vi "Value_JSON.vi"(0 "Data JSON":string, 5 "Type":string, 7 "Size data":string, 9 "Hexa":string, 11 "error in":errorcluster) -> (4 "Value_string":string, 8 "Hexa value":string, 15 "error IO":errorcluster)   [LabVIEW 2021]
uses:
  <vilib>/JDP Science/JSONtext/String Subset.vi
  <vilib>/JDP Science/JSONtext/support/Strip Quotes and Unescape.vi
  <vilib>/JDP Science/JSONtext/support/Unescape JSON string.vi
  <vilib>/JDP Science/JSONtext/Parsing/Parse Full Path or Item Name.vi
  <vilib>/JDP Science/JSONtext/Offset/Find Item Locations by Path.vi
  <vilib>/JDP Science/JSONtext/JSONtext.lvlib
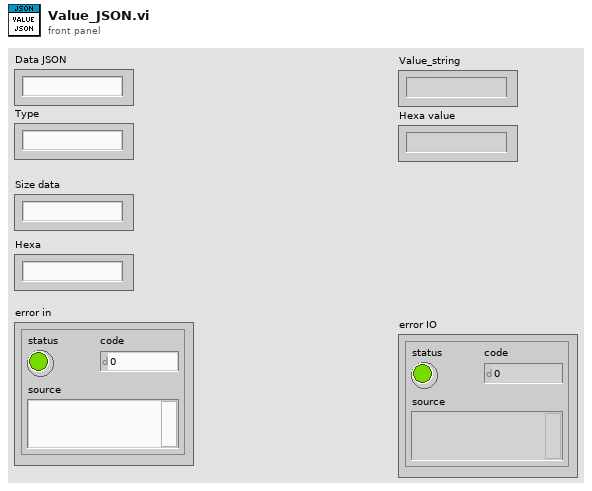
[diagram p1: front panel]
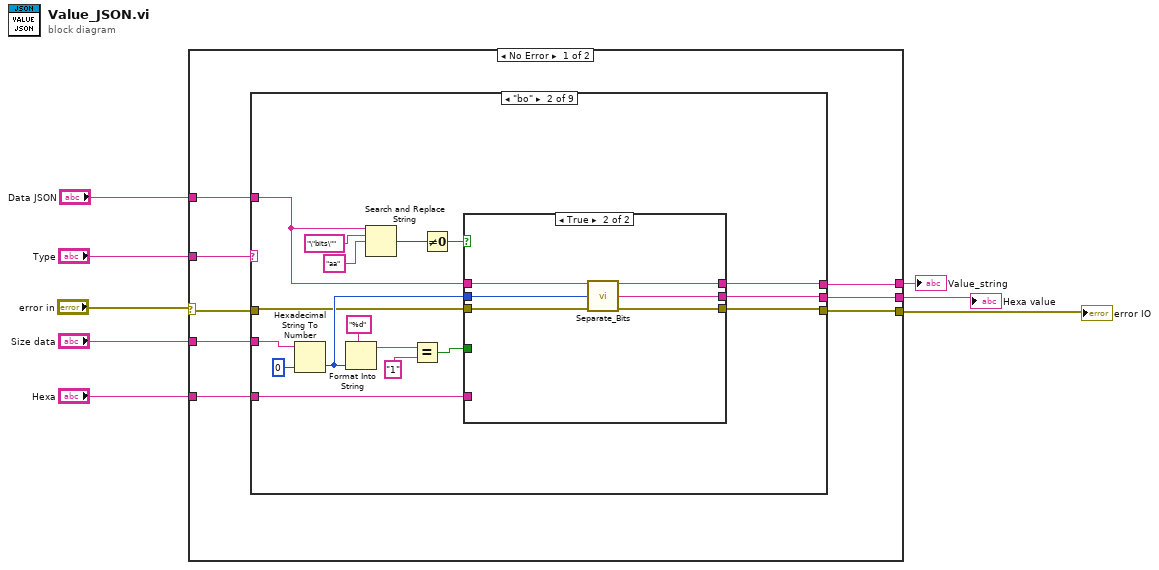
[diagram p0: block diagram]
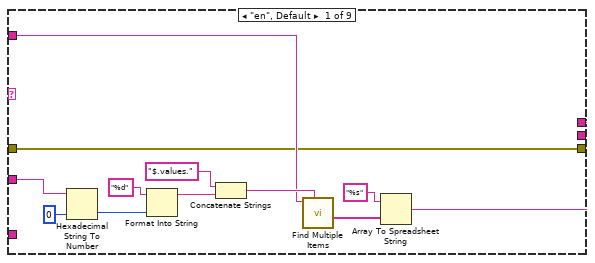
[diagram p2: hidden frame]
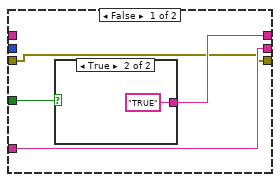
[diagram p3: hidden frame]
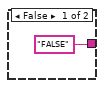
[diagram p4: hidden frame]
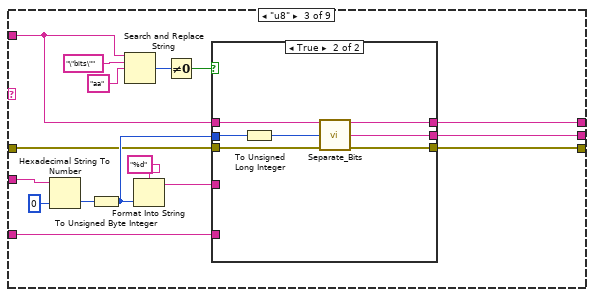
[diagram p5: hidden frame]
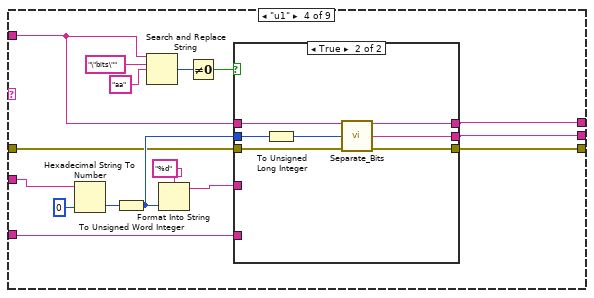
[diagram p7: hidden frame]
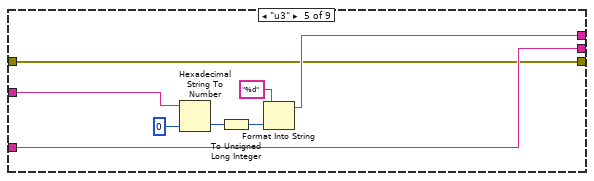
[diagram p9: hidden frame]
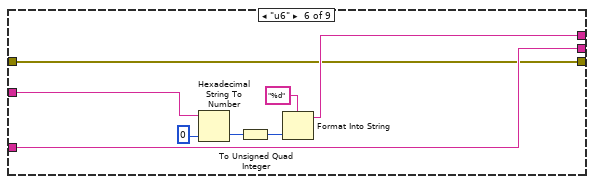
[diagram p10: hidden frame]
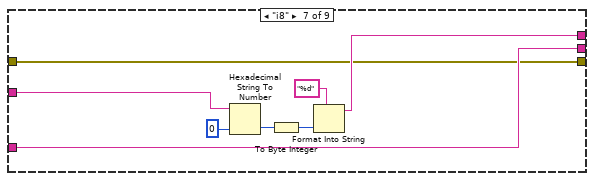
[diagram p11: hidden frame]
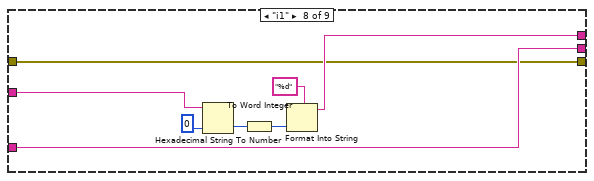
[diagram p12: hidden frame]
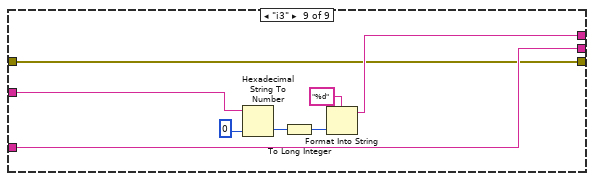
[diagram p13: hidden frame]
diagram:
  n1 = case shown="No Error" "error in" {
    selector: "error in" -> [w12 w150]
    tunnel: "Data JSON" -> [w16 _]
    tunnel: "Size data" -> [w15 _]
    tunnel: "Type" -> [w14 _]
    tunnel: "Hexa" -> [w13 _]
    tunnel: [w11 w150] -> w1
    tunnel: [w10 _] -> w2
    tunnel: [w9 _] -> w3
    frame No Error {
      n2 = case shown="\"bo\"" w14 {
        tunnel: w15 -> [w22 w44 w66 w89 w113 w121 w129 w137 w145]
        tunnel: [w19 w34 w64 w87 w112 w120 w128 w136 w144] -> w9
        tunnel: [_ w33 w61 w86 w111 w119 w127 w135 w143] -> w10
        tunnel: w13 -> [_ w32 w62 w90 w111 w119 w127 w135 w143]
        tunnel: w16 -> [w18 w36 w63 w88 _ _ _ _ _]
        tunnel: w12 -> [w17 w30 w59 w85 w110 w118 w126 w134 w142]
        tunnel: [w17 w29 w58 w84 w110 w118 w126 w134 w142] -> w11
        frame "en", Default {
          n3 = Hexadecimal String To Number(string=w22, default (0uL)=u32 0 ("default (0 U32)")) -> (number=w28:u32)  [unwired: 1 in, 1 out]
          n4 = Format Into String(format string="%d", w28) -> (resulting string=w25:string)  [unwired: 2 in, 1 out]
          n5 = Concatenate Strings("$.values." ("string"), w25) -> (w24:string)
          n6 = call <vilib>:"Find Multiple Items.vi"("$Path or Item Name"=w24, "JSON"=w18) -> ("<JSON>"=w20:string[])  [unwired: 6 in, 3 out]
          n7 = Array To Spreadsheet String(array=w20, 3:"%s" ("format string")) -> (spreadsheet string=w19:string)  [unwired: 1 in]
        }
        frame "bo" {
          n8 = Hexadecimal String To Number(string=w44, default (0uL)=u32 0 ("default (0 U32)")) -> (number=w31:u32)  [unwired: 1 in, 1 out]
          n9 = Format Into String(format string="%d", w31) -> (resulting string=w43:string)  [unwired: 2 in, 1 out]
          n10 = Search and Replace String(input string=w36, search string="\"bits\"", replace string="aa" ("replace string (\"\")")) -> (number of replacements=w38:i32)  [unwired: 5 in, 3 out]
          n11 = Equal?(x=w43, y="1") -> (x = y?=w35:bool)
          n12 = Not Equal To 0?(x=w38) -> (x != 0?=w37:bool)
          n13 = case shown="True" w37 {
            tunnel: [w48 w55] -> w34
            tunnel: w36 -> [_ w57]
            tunnel: [w47 w54] -> w33
            tunnel: w35 -> [w49 _]
            tunnel: w32 -> [w47 _]
            tunnel: w31 -> [_ w56]
            tunnel: w30 -> [w46 w53]
            tunnel: [w46 w52] -> w29
            frame False {
              n14 = case shown="True" w49 {
                tunnel: ["FALSE" "TRUE"] -> w48
                frame False {
                }
                frame True {
                }
              }
            }
            frame True {
              n15 = call "Separate_Bits.vi"("JSON"=w57, "int size number"=w56, "error in"=w53) -> ("Value_string"=w55:string, "hex_data"=w54:string, "error out"=w52:errorcluster)  [unwired: 10 in]
            }
          }
        }
        frame "u8" {
          n16 = Hexadecimal String To Number(string=w66, default (0uL)=u32 0 ("default (0 U32)")) -> (number=w71:u32)  [unwired: 1 in, 1 out]
          n17 = To Unsigned Byte Integer(number=w71) -> (unsigned 8bit integer=w60:u8)
          n18 = Search and Replace String(input string=w63, search string="\"bits\"", replace string="aa" ("replace string (\"\")")) -> (number of replacements=w68:i32)  [unwired: 5 in, 3 out]
          n19 = Format Into String(format string="%d", w60) -> (resulting string=w65:string)  [unwired: 2 in, 1 out]
          n20 = Not Equal To 0?(x=w68) -> (x != 0?=w67:bool)
          n21 = case shown="True" w67 {
            tunnel: [w76 w80] -> w64
            tunnel: w65 -> [w76 _]
            tunnel: w63 -> [_ w83]
            tunnel: w62 -> [w75 _]
            tunnel: [w75 w79] -> w61
            tunnel: w60 -> [_ w82]
            tunnel: w59 -> [w74 w78]
            tunnel: [w74 w77] -> w58
            frame False {
            }
            frame True {
              n22 = To Unsigned Long Integer(number=w82) -> (unsigned 32bit integer=w81:u32)
              n23 = call "Separate_Bits.vi"("JSON"=w83, "int size number"=w81, "error in"=w78) -> ("Value_string"=w80:string, "hex_data"=w79:string, "error out"=w77:errorcluster)  [unwired: 10 in]
            }
          }
        }
        frame "u1" {
          n24 = Hexadecimal String To Number(string=w89, default (0uL)=u32 0 ("default (0 U32)")) -> (number=w95:u32)  [unwired: 1 in, 1 out]
          n25 = To Unsigned Word Integer(number=w95) -> (unsigned 16bit integer=w99:u16)
          n26 = Search and Replace String(input string=w88, search string="\"bits\"", replace string="aa" ("replace string (\"\")")) -> (number of replacements=w96:i32)  [unwired: 5 in, 3 out]
          n27 = Format Into String(format string="%d", w99) -> (resulting string=w98:string)  [unwired: 2 in, 1 out]
          n28 = Not Equal To 0?(x=w96) -> (x != 0?=w97:bool)
          n29 = case shown="True" w97 {
            tunnel: [w102 w106] -> w87
            tunnel: w98 -> [w102 _]
            tunnel: w88 -> [_ w109]
            tunnel: w90 -> [w101 _]
            tunnel: [w101 w105] -> w86
            tunnel: w99 -> [_ w108]
            tunnel: w85 -> [w100 w104]
            tunnel: [w100 w103] -> w84
            frame False {
            }
            frame True {
              n30 = To Unsigned Long Integer(number=w108) -> (unsigned 32bit integer=w107:u32)
              n31 = call "Separate_Bits.vi"("JSON"=w109, "int size number"=w107, "error in"=w104) -> ("Value_string"=w106:string, "hex_data"=w105:string, "error out"=w103:errorcluster)  [unwired: 10 in]
            }
          }
        }
        frame "u3" {
          n32 = Hexadecimal String To Number(string=w113, default (0uL)=u32 0 ("default (0 U32)")) -> (number=w116:u32)  [unwired: 1 in, 1 out]
          n33 = To Unsigned Long Integer(number=w116) -> (unsigned 32bit integer=w117:u32)
          n34 = Format Into String(format string="%d", w117) -> (resulting string=w112:string)  [unwired: 2 in, 1 out]
        }
        frame "u6" {
          n35 = Hexadecimal String To Number(string=w121, default (0uL)=u32 0 ("default (0 U32)")) -> (number=w124:u32)  [unwired: 1 in, 1 out]
          n36 = To Unsigned Quad Integer(1:w124) -> (0:w125:u64)
          n37 = Format Into String(format string="%d", w125) -> (resulting string=w120:string)  [unwired: 2 in, 1 out]
        }
        frame "i8" {
          n38 = Hexadecimal String To Number(string=w129, default (0uL)=u32 0 ("default (0 U32)")) -> (number=w132:u32)  [unwired: 1 in, 1 out]
          n39 = To Byte Integer(number=w132) -> (8bit integer=w133:i8)
          n40 = Format Into String(format string="%d", w133) -> (resulting string=w128:string)  [unwired: 2 in, 1 out]
        }
        frame "i1" {
          n41 = Hexadecimal String To Number(string=w137, default (0uL)=u32 0 ("default (0 U32)")) -> (number=w140:u32)  [unwired: 1 in, 1 out]
          n42 = To Word Integer(number=w140) -> (16bit integer=w141:i16)
          n43 = Format Into String(format string="%d", w141) -> (resulting string=w136:string)  [unwired: 2 in, 1 out]
        }
        frame "i3" {
          n44 = Hexadecimal String To Number(string=w145, default (0uL)=u32 0 ("default (0 U32)")) -> (number=w148:u32)  [unwired: 1 in, 1 out]
          n45 = To Long Integer(number=w148) -> (32bit integer=w149:i32)
          n46 = Format Into String(format string="%d", w149) -> (resulting string=w144:string)  [unwired: 2 in, 1 out]
        }
      }
    }
    frame Error {
    }
  }
  "Value_string" <- w3
  "Hexa value" <- w2
  "error IO" <- w1
